vi "PLC RECIPE UPLOAD TESTED.vi"() -> ()   [LabVIEW 2017]
uses:
  <vilib>/ethernetip/ethernetip.llb/EthernetIP SLC500 Read Integer.vi
  <vilib>/ethernetip/ethernetip.lvlib
panel:
  out "error in 2":errorcluster
  out "element 2":i16
  out "Data 2":i16[](array[numeric])
  out "Data":i16[](array[numeric])
  out "element":i16
  out "error in":errorcluster
  # "YEAR\nMONTH\nDAY\nHOUR\nMINUTE\nRECIPENUMBER\nPROD QUNTY"
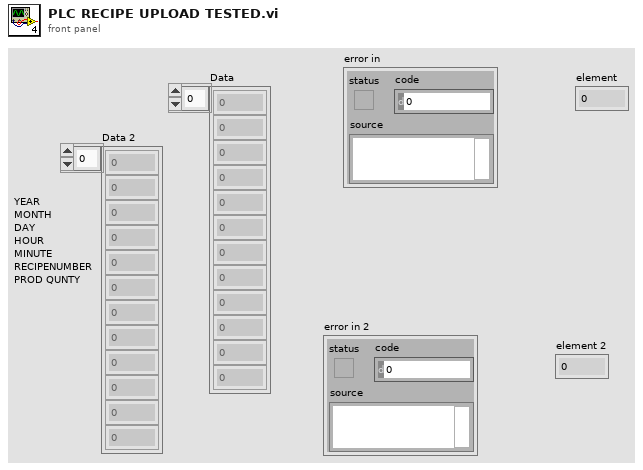
[diagram p1: front panel]
types:
  T1 = typedef "ethernetip.lvlib/ethernetip.ctl" = refnum<k21>
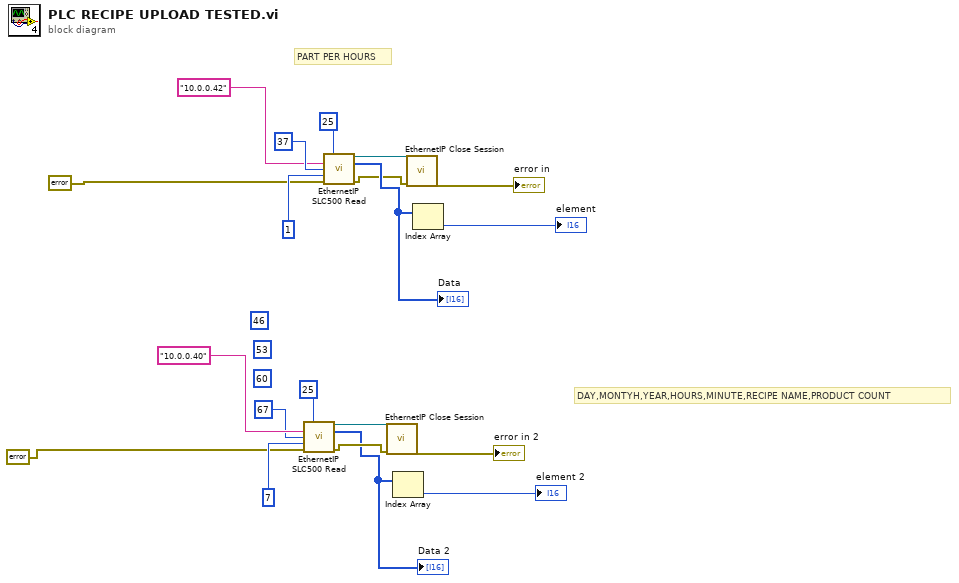
[diagram p0: block diagram]
diagram:
  (unwired) u16 60 ("Element Number")
  (unwired) u16 53 ("Element Number")
  (unwired) u16 46 ("Element Number")
  # "DAY,MONTYH,YEAR,HOURS,MINUTE,RECIPE NAME,PRODUCT COUNT"
  # "PART PER HOURS"
  n1 = call-poly <vilib>:"EthernetIP SLC500 Read.vi"("File Number"=u16 25, "Network Path"="10.0.0.40", "Element Number"=u16 67, "Number of Elements"=u32 7, "error in"=errorcluster {"status"=FALSE, "code"=0, "source"=""}) -> ("Session out"=w6:T1, "Data"=w2:i16[], "error out"=w5:errorcluster)  [unwired: 8 in]
  "Data 2" <- w2
  n2 = call-poly <vilib>:"EthernetIP SLC500 Read.vi"("File Number"=u16 25, "Network Path"="10.0.0.42", "Element Number"=u16 37, "Number of Elements"=u32 1, "error in"=errorcluster {"status"=FALSE, "code"=0, "source"=""}) -> ("Session out"=w16:T1, "Data"=w20:i16[], "error out"=w17:errorcluster)  [unwired: 8 in]
  "Data" <- w20
  n3 = call <vilib>:"EthernetIP Close Session.vi"("error in"=w5, "Session in"=w6) -> ("error out"=→"error in 2":errorcluster)  [unwired: 9 in]
  n4 = Index Array(array=w2) -> (element=→"element 2":i16)  [unwired: 1 in]
  n5 = call <vilib>:"EthernetIP Close Session.vi"("error in"=w17, "Session in"=w16) -> ("error out"=→"error in":errorcluster)  [unwired: 9 in]
  n6 = Index Array(array=w20) -> (element=→"element":i16)  [unwired: 1 in]
